vi "MonitorTemperatureChange.vi"(8 "error in (no error)":errorcluster, 10 "Array Out":waveform(dbl)[](array[waveform]), 11 "RoomAlert in":refnum<class "RoomAlert.lvclass">) -> (0 "error out":errorcluster, 2 "TempChangeExceedLimits":bool, 3 "RoomAlert out":refnum<class "RoomAlert.lvclass">)   [LabVIEW 2018, in "SensorPlugins.lvlib" / "RoomAlert.lvclass"]
uses:
  RoomAlert.lvclass
  <vilib>/Utility/error.llb/Error Cluster From Error Code.vi
  <vilib>/ErrorRing/Error Ring.xnode
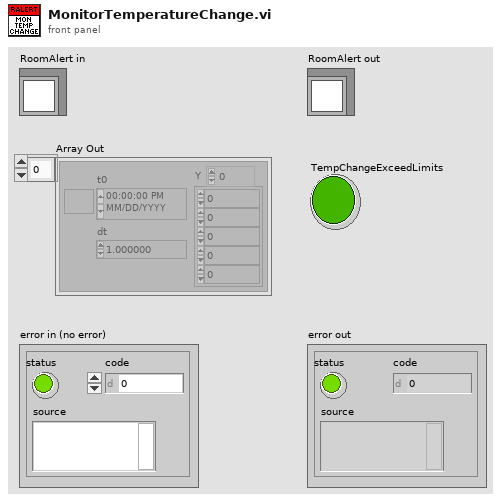
[diagram p1: front panel]
types:
  T1 = typedef "SensorPlugins.lvlib/RoomAlert.lvclass/MeasurementControls.ctl" = cluster{"Measurement RefreshTime (ms)":u32, "Measurement Name":string, "Timeout(ms)":i32, "Amber Warning Light Configuration":cluster{"Warning Temperture (Degrees C)":dbl, "Temperature Delta (Degrees C/Minute)":dbl, "Time Window (Minutes)":dbl}}
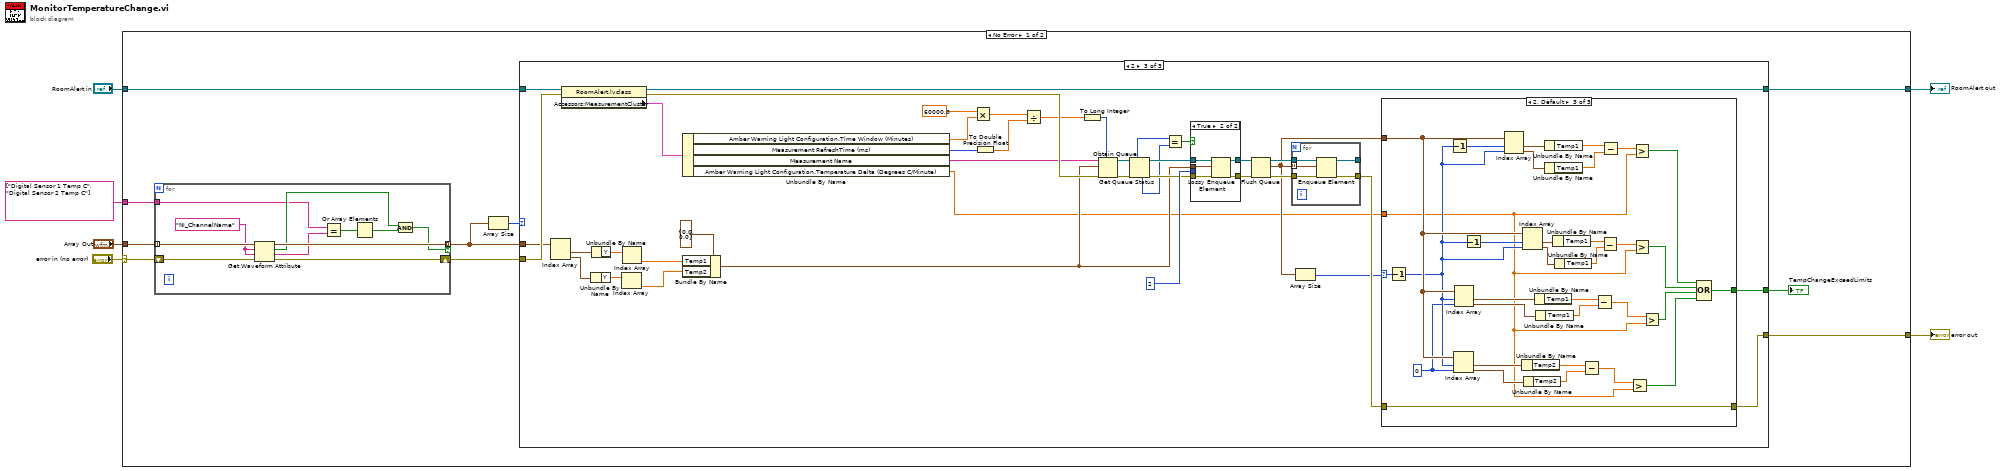
[diagram p0: block diagram]
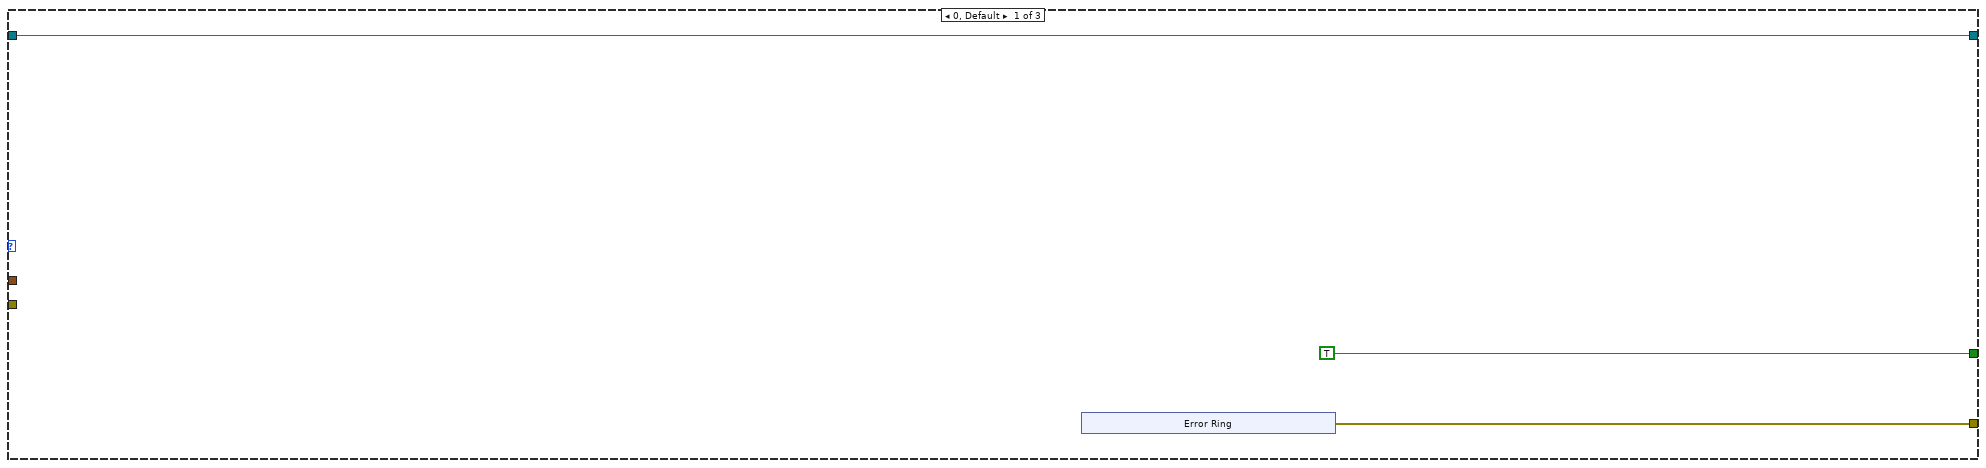
[diagram p2: hidden frame]
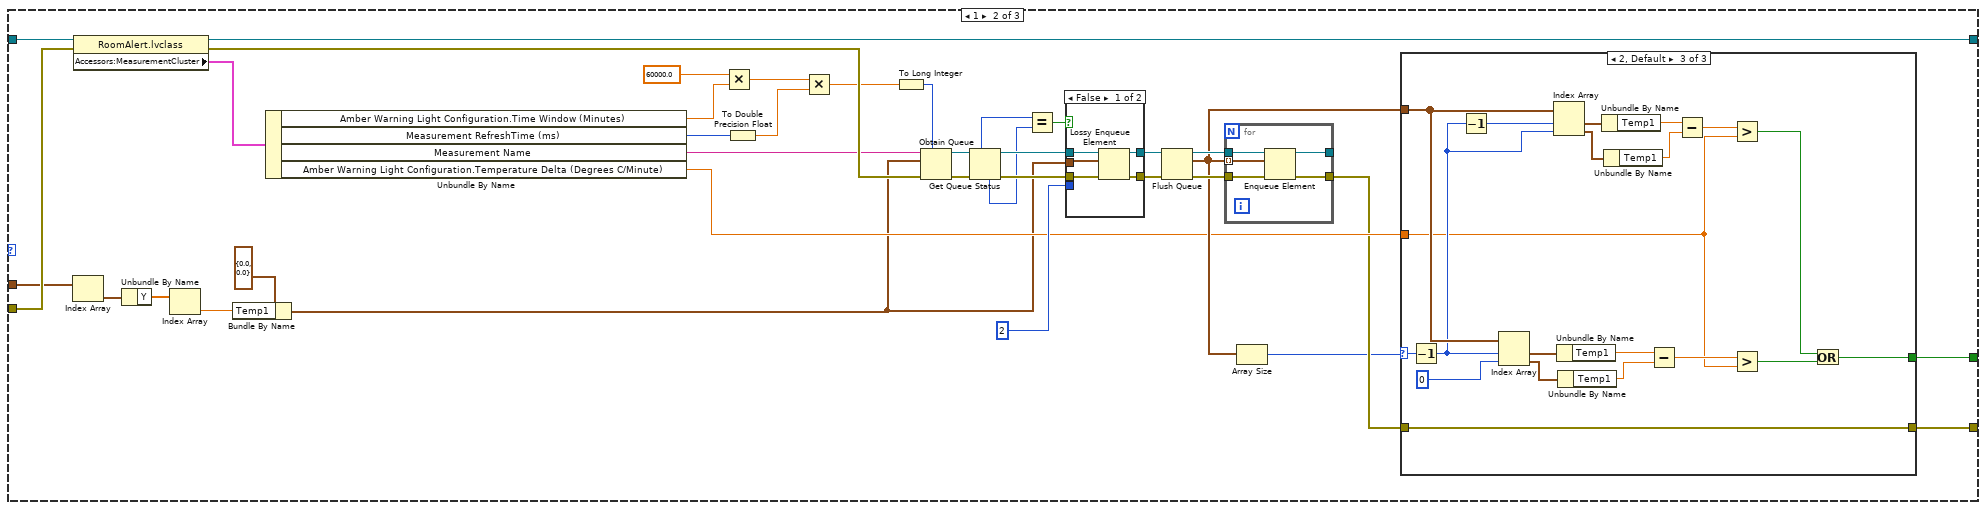
[diagram p3: hidden frame]
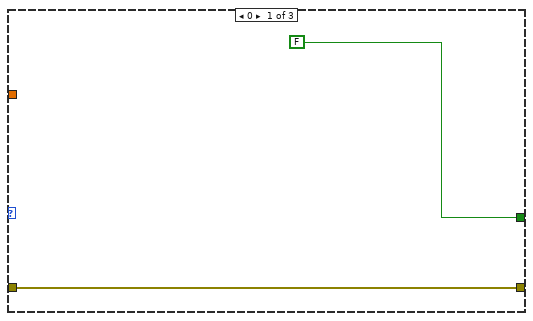
[diagram p4: hidden frame]
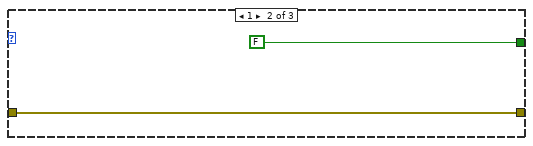
[diagram p5: hidden frame]
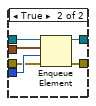
[diagram p6: hidden frame]
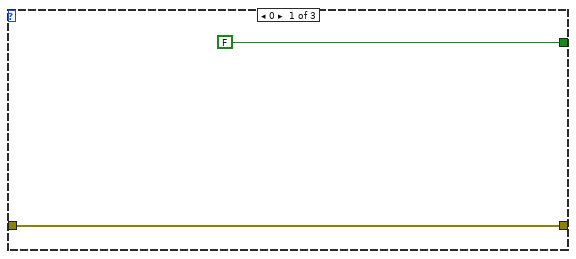
[diagram p7: hidden frame]
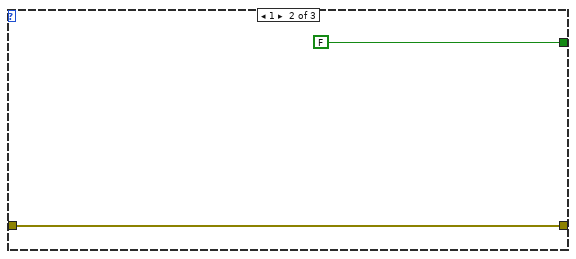
[diagram p8: hidden frame]
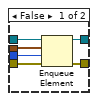
[diagram p9: hidden frame]
diagram:
  n1 = case shown="No Error" "error in (no error)" {
    selector: "error in (no error)" -> [w12 w207]
    tunnel: [w14 w207] -> w5
    tunnel: [w15 w206] -> w3
    tunnel: "RoomAlert in" -> [w16 w206]
    tunnel: "Array Out" -> [w13 _]
    tunnel: string[] ["Digital Sensor 1 Temp C", "Digital Sensor 2 Temp C"] -> [w7 _]
    frame No Error {
      n2 = for {
        tunnel: w13 -> [w27] mode=indexing
        tunnel: [w24] -> w10 mode=indexing if=w19
        shift-right: [w18] -> w11
        shift-left: w12 -> [w26]
        tunnel: w7 -> [w17]
        w25 = "NI_ChannelName" ("name")
        n3 = Get Waveform Attribute(4:w26, 5:w25, 6:w25, 7:w27) -> (0:w18:errorcluster, 1:w22:string, 2:w23:bool, 3:w24:waveform(dbl))
        n4 = Equal?(x=w17, y=w22) -> (x = y?=w21:bool[])
        n5 = Or Array Elements(Boolean array=w21) -> (logical OR=w20:bool)
        n6 = Compound Arithmetic op=AND(w23, w20) -> (w19:bool)
      }
      n7 = Array Size(array=w10) -> (size(s)=w9:i32)
      n8 = case shown="2" w9 {
        tunnel: w16 -> [w30 w72 w152]
        tunnel: [w30 w71 w151] -> w15
        tunnel: [w29 w50 w118] -> w14
        tunnel: w11 -> [_ w44 w128]
        tunnel: w10 -> [_ w42 w127]
        tunnel: [TRUE w43 w117] -> w8
        frame 0, Default {
          n9 = xnode "Error Ring"() -> ("error out"=w29:errorcluster)
        }
        frame 1 {
          n10 = Index Array(array=w42) -> (element=w40:waveform(dbl))  [unwired: 1 in]
          n11 = property class="RoomAlert.lvclass"(reference=w72, error in=w44) -> (reference out=w71:refnum<class "RoomAlert.lvclass">, error out=w70:errorcluster, "Accessors:MeasurementCluster"=w68:T1)
          n12 = Unbundle By Name(w40) -> ("Y"=w41:dbl[])
          n13 = Index Array(array=w41) -> (element=w38:dbl)  [unwired: 1 in]
          n14 = Bundle By Name(cluster=cluster{"Temp1":dbl, "Temp2":dbl} {"Temp1"=0.0, "Temp2"=0.0} ("Cluster"), "Temp1"=w38) -> (w37:cluster{"Temp1":dbl, "Temp2":dbl})
          n15 = Unbundle By Name(w68) -> ("Amber Warning Light Configuration.Time Window (Minutes)"=w53:dbl, "Measurement RefreshTime (ms)"=w46:u32, "Measurement Name"=w69:string, "Amber Warning Light Configuration.Temperature Delta (Degrees C/Minute)"=w52:dbl)
          n16 = Multiply(x=60000.0, y=w53) -> (x*y=w67:dbl)
          n17 = To Double Precision Float(number=w46) -> (double precision float=w45:dbl)
          n18 = Multiply(x=w67, y=w45) -> (x*y=w49:dbl)
          n19 = To Long Integer(number=w49) -> (32bit integer=w48:i32)
          n20 = Obtain Queue(max queue size (-1, unlimited)=w48, name (unnamed)=w69, element data type=w37, error in (no error)=w70) -> (queue out=w61:refnum<queue>, error out=w63:errorcluster)  [unwired: 1 in, 1 out]
          n21 = Get Queue Status(queue=w61, error in (no error)=w63) -> (queue out=w60:refnum<queue>, max queue size=w58:i32, error out=w62:errorcluster, # elements in queue=w59:i32)  [unwired: 1 in, 4 out]
          n22 = Equal?(x=w58, y=w59) -> (x = y?=w57:bool)
          n23 = case shown="False" w57 {
            tunnel: w37 -> [w102 w112]
            tunnel: [w106 w111] -> w66
            tunnel: [w103 w110] -> w65
            tunnel: 2 ("timeout in ms (-1)") -> [_ w109]
            tunnel: w62 -> [w105 w108]
            tunnel: w60 -> [w104 w107]
            frame False {
              n24 = Lossy Enqueue Element(queue=w104, element=w102, error in (no error)=w105) -> (queue out=w103:refnum<queue>, error out=w106:errorcluster)  [unwired: 2 out]
            }
            frame True {
              n25 = Enqueue Element(queue=w107, element=w112, timeout in ms (-1)=w109, error in (no error)=w108) -> (queue out=w110:refnum<queue>, error out=w111:errorcluster)  [unwired: 1 out]
            }
          }
          n26 = Flush Queue(queue=w65, error in (no error)=w66) -> (queue out=w56:refnum<queue>, remaining elements=w54:cluster{"Temp1":dbl, "Temp2":dbl}[], error out=w55:errorcluster)
          n27 = for {
            tunnel: w54 -> [w77] mode=indexing
            tunnel: w56 -> [w76]
            tunnel: w55 -> [w75]
            tunnel: [w74] -> w51
            tunnel: [w73] -> _
            n28 = Enqueue Element(queue=w76, element=w77, error in (no error)=w75) -> (queue out=w73:refnum<queue>, error out=w74:errorcluster)  [unwired: 1 in, 1 out]
          }
          n29 = Array Size(array=w54) -> (size(s)=w36:i32)
          n30 = case shown="2, Default" w36 {
            selector: w36 -> [_ _ w90]
            tunnel: w54 -> [_ _ w98]
            tunnel: w52 -> [_ _ w83]
            tunnel: w51 -> [w79 w80 w101]
            tunnel: [w79 w80 w101] -> w50
            tunnel: [FALSE FALSE w92] -> w43
            frame 0 {
            }
            frame 1 {
            }
            frame 2, Default {
              n31 = Decrement(x=w90) -> (x-1=w84:i32)
              n32 = Decrement(x=w84) -> (x-1=w85:i32)
              n33 = Index Array(array=w98, index #1=w84, index #2=0 ("index")) -> (element #1=w99:cluster{"Temp1":dbl, "Temp2":dbl}, element #2=w97:cluster{"Temp1":dbl, "Temp2":dbl})
              n34 = Index Array(array=w98, index #1=w85, index #2=w84) -> (element #1=w100:cluster{"Temp1":dbl, "Temp2":dbl}, element #2=w89:cluster{"Temp1":dbl, "Temp2":dbl})
              n35 = Unbundle By Name(w99) -> ("Temp1"=w95:dbl)
              n36 = Unbundle By Name(w97) -> ("Temp1"=w94:dbl)
              n37 = Unbundle By Name(w100) -> ("Temp1"=w87:dbl)
              n38 = Unbundle By Name(w89) -> ("Temp1"=w86:dbl)
              n39 = Subtract(x=w95, y=w94) -> (x-y=w91:dbl)
              n40 = Subtract(x=w87, y=w86) -> (x-y=w88:dbl)
              n41 = Greater?(x=w88, y=w83) -> (0:w82:bool)
              n42 = Greater?(x=w91, y=w83) -> (0:w93:bool)
              n43 = Or(x=w82, y=w93) -> (x .or. y?=w92:bool)
            }
          }
        }
        frame 2 {
          n44 = Index Array(array=w127) -> (element #1=w125:waveform(dbl), element #2=w123:waveform(dbl))  [unwired: 2 in]
          n45 = property class="RoomAlert.lvclass"(reference=w152, error in=w128) -> (reference out=w151:refnum<class "RoomAlert.lvclass">, error out=w150:errorcluster, "Accessors:MeasurementCluster"=w148:T1)
          n46 = Unbundle By Name(w123) -> ("Y"=w124:dbl[])
          n47 = Unbundle By Name(w125) -> ("Y"=w126:dbl[])
          n48 = Index Array(array=w124) -> (element=w120:dbl)  [unwired: 1 in]
          n49 = Index Array(array=w126) -> (element=w121:dbl)  [unwired: 1 in]
          n50 = Unbundle By Name(w148) -> ("Amber Warning Light Configuration.Time Window (Minutes)"=w134:dbl, "Measurement RefreshTime (ms)"=w130:u32, "Measurement Name"=w149:string, "Amber Warning Light Configuration.Temperature Delta (Degrees C/Minute)"=w114:dbl)
          n51 = Bundle By Name(cluster=cluster{"Temp1":dbl, "Temp2":dbl} {"Temp1"=0.0, "Temp2"=0.0} ("Cluster"), "Temp1"=w121, "Temp2"=w120) -> (w119:cluster{"Temp1":dbl, "Temp2":dbl})
          n52 = Multiply(x=60000.0, y=w134) -> (x*y=w147:dbl)
          n53 = To Double Precision Float(number=w130) -> (double precision float=w129:dbl)
          n54 = Divide(x=w147, y=w129) -> (x/y=w133:dbl)
          n55 = To Long Integer(number=w133) -> (32bit integer=w132:i32)
          n56 = Obtain Queue(max queue size (-1, unlimited)=w132, name (unnamed)=w149, element data type=w119, error in (no error)=w150) -> (queue out=w141:refnum<queue>, error out=w143:errorcluster)  [unwired: 1 in, 1 out]
          n57 = Get Queue Status(queue=w141, error in (no error)=w143) -> (queue out=w140:refnum<queue>, max queue size=w138:i32, error out=w142:errorcluster, # elements in queue=w139:i32)  [unwired: 1 in, 4 out]
          n58 = Equal?(x=w138, y=w139) -> (x = y?=w137:bool)
          n59 = case shown="True" w137 {
            tunnel: w119 -> [w200 w201]
            tunnel: [w199 w205] -> w146
            tunnel: [w198 w202] -> w145
            tunnel: 2 ("timeout in ms (-1)") -> [w197 _]
            tunnel: w142 -> [w196 w204]
            tunnel: w140 -> [w195 w203]
            frame False {
              n60 = Enqueue Element(queue=w195, element=w200, timeout in ms (-1)=w197, error in (no error)=w196) -> (queue out=w198:refnum<queue>, error out=w199:errorcluster)  [unwired: 1 out]
            }
            frame True {
              n61 = Lossy Enqueue Element(queue=w203, element=w201, error in (no error)=w204) -> (queue out=w202:refnum<queue>, error out=w205:errorcluster)  [unwired: 2 out]
            }
          }
          n62 = Flush Queue(queue=w145, error in (no error)=w146) -> (queue out=w136:refnum<queue>, remaining elements=w115:cluster{"Temp1":dbl, "Temp2":dbl}[], error out=w135:errorcluster)
          n63 = for {
            tunnel: w115 -> [w194] mode=indexing
            tunnel: w136 -> [w193]
            tunnel: w135 -> [w192]
            tunnel: [w191] -> w116
            tunnel: [w190] -> _
            n64 = Enqueue Element(queue=w193, element=w194, error in (no error)=w192) -> (queue out=w190:refnum<queue>, error out=w191:errorcluster)  [unwired: 1 in, 1 out]
          }
          n65 = Array Size(array=w115) -> (size(s)=w113:i32)
          n66 = case shown="2, Default" w113 {
            selector: w113 -> [_ _ w176]
            tunnel: w115 -> [_ _ w161]
            tunnel: w114 -> [_ _ w159]
            tunnel: w116 -> [w154 w156 w189]
            tunnel: [w154 w156 w189] -> w118
            tunnel: [FALSE FALSE w183] -> w117
            frame 0 {
            }
            frame 1 {
            }
            frame 2, Default {
              w157 = 0 ("index")
              n67 = Decrement(x=w176) -> (x-1=w160:i32)
              n68 = Decrement(x=w160) -> (x-1=w169:i32)
              n69 = Index Array(array=w161, index #1=w160, index #2=w157) -> (element #1=w177:cluster{"Temp1":dbl, "Temp2":dbl}, element #2=w178:cluster{"Temp1":dbl, "Temp2":dbl})
              n70 = Index Array(array=w161, index #1=w160, index #2=w157) -> (element #1=w188:cluster{"Temp1":dbl, "Temp2":dbl}, element #2=w187:cluster{"Temp1":dbl, "Temp2":dbl})
              n71 = Decrement(x=w160) -> (x-1=w167:i32)
              n72 = Index Array(array=w161, index #1=w169, index #2=w160) -> (element #1=w174:cluster{"Temp1":dbl, "Temp2":dbl}, element #2=w173:cluster{"Temp1":dbl, "Temp2":dbl})
              n73 = Unbundle By Name(w177) -> ("Temp2"=w179:dbl)
              n74 = Index Array(array=w161, index #1=w167, index #2=w160) -> (element #1=w162:cluster{"Temp1":dbl, "Temp2":dbl}, element #2=w163:cluster{"Temp1":dbl, "Temp2":dbl})
              n75 = Unbundle By Name(w178) -> ("Temp2"=w180:dbl)
              n76 = Unbundle By Name(w188) -> ("Temp1"=w186:dbl)
              n77 = Unbundle By Name(w187) -> ("Temp1"=w185:dbl)
              n78 = Unbundle By Name(w174) -> ("Temp1"=w171:dbl)
              n79 = Unbundle By Name(w173) -> ("Temp1"=w170:dbl)
              n80 = Unbundle By Name(w162) -> ("Temp1"=w165:dbl)
              n81 = Unbundle By Name(w163) -> ("Temp1"=w166:dbl)
              n82 = Subtract(x=w179, y=w180) -> (x-y=w181:dbl)
              n83 = Subtract(x=w186, y=w185) -> (x-y=w182:dbl)
              n84 = Subtract(x=w165, y=w166) -> (x-y=w164:dbl)
              n85 = Subtract(x=w171, y=w170) -> (x-y=w172:dbl)
              n86 = Greater?(x=w181, y=w159) -> (0:w175:bool)
              n87 = Greater?(x=w172, y=w159) -> (0:w168:bool)
              n88 = Greater?(x=w164, y=w159) -> (0:w158:bool)
              n89 = Greater?(x=w182, y=w159) -> (0:w184:bool)
              n90 = Compound Arithmetic op=OR(w168, w158, w184, w175) -> (w183:bool)
            }
          }
        }
      }
      "TempChangeExceedLimits" <- w8
    }
    frame Error {
    }
  }
  "error out" <- w5
  "RoomAlert out" <- w3
